vi "test_c.vi"() -> ()   [LabVIEW 2026]
uses:
  variant_test.dll
panel:
  out "Array 2":errorcluster[](array[cluster])
  out "Array":i32[](array[numeric])
  out "return type 2":i32
  out "result 2":i32
  out "variant 2":variant
  out "error out 2":errorcluster
  out "error out":errorcluster
  out "variant":variant
  out "result":i32
  out "return type":i32
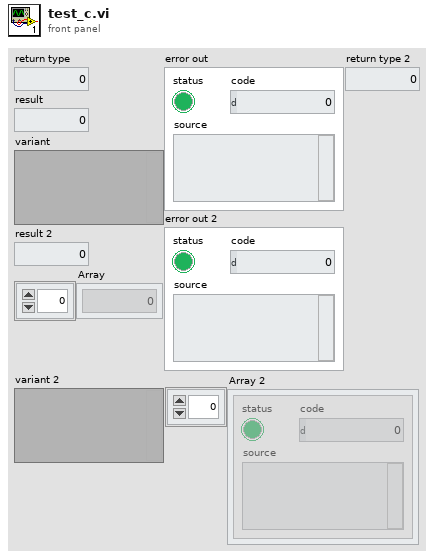
[diagram p1: front panel]
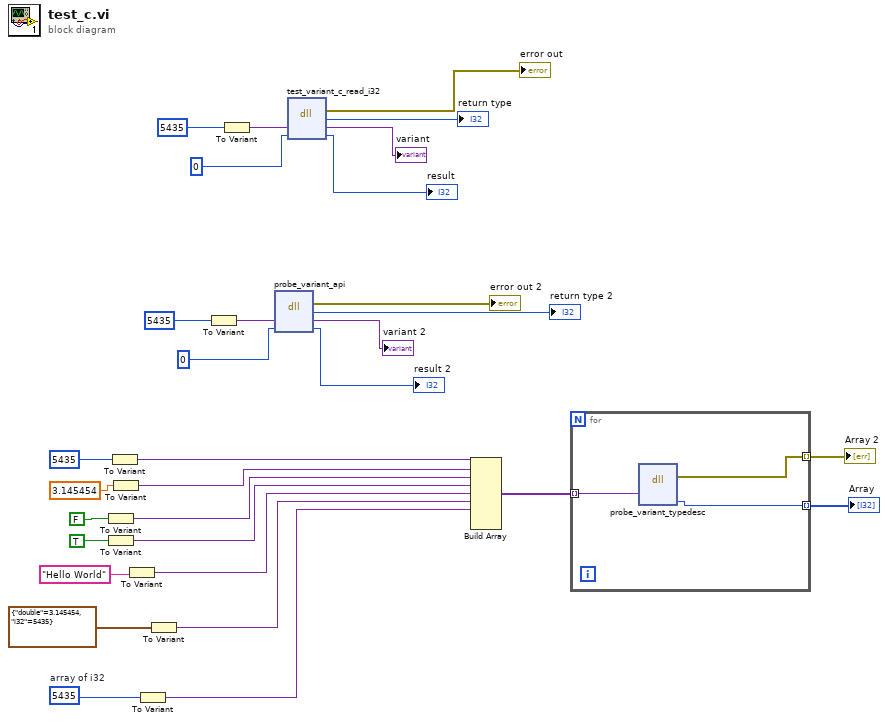
[diagram p0: block diagram]
diagram:
  w5 = 5435  # array of i32
  n1 = To Variant(anything=FALSE) -> (Variant=w12:variant)
  n2 = To Variant(anything=TRUE) -> (Variant=w11:variant)
  n3 = To Variant(anything=5435) -> (Variant=w16:variant)
  n4 = To Variant(anything=3.145454) -> (Variant=w14:variant)
  n5 = To Variant(anything="Hello World") -> (Variant=w8:variant)
  n6 = To Variant(anything=w5) -> (Variant=w4:variant)
  n7 = To Variant(anything=cluster{"double":dbl, "i32":i32} {"double"=3.145454, "i32"=5435}) -> (Variant=w6:variant)
  n8 = To Variant(anything=5435) -> (Variant=w22:variant)
  n9 = To Variant(anything=5435) -> (Variant=w27:variant)
  n10 = dll-call lib="C:/Git/Rust-LabVIEW-Interop/variant_test.dll" fn="probe_variant_api"("variant"=w22, "result"=0) -> (error out=→"error out 2":errorcluster, "return type"=→"return type 2":i32, "variant"=→"variant 2":variant, "result"=→"result 2":i32)  [unwired: 3 in, 1 out]
  n11 = dll-call lib="C:/Git/Rust-LabVIEW-Interop/variant_test.dll" fn="test_variant_c_read_i32"("variant"=w27, "result"=0) -> (error out=→"error out":errorcluster, "return type"=→"return type":i32, "variant"=→"variant":variant, "result"=→"result":i32)  [unwired: 3 in, 1 out]
  n12 = Build Array(w16, w14, w12, w11, w8, w6, w4) -> (w3:variant[])  [unwired: 2 in]
  n13 = for {
    tunnel: w3 -> [w34] mode=indexing
    tunnel: [w33] -> w2 mode=indexing
    tunnel: [w32] -> w1 mode=indexing
    n14 = dll-call lib="C:/Git/Rust-LabVIEW-Interop/variant_test.dll" fn="probe_variant_typedesc"("variant"=w34) -> (error out=w32:errorcluster, "result"=w33:i32)  [unwired: 6 in, 1 out]
  }
  "Array" <- w2
  "Array 2" <- w1
